vi "Magnet Test Communications.vi"(8 "error in (no error)":errorcluster, 11 "VISA resource name in":refnum<visa-resource-name>) -> (0 "error out":errorcluster, 3 "VISA resource name out":refnum<visa-resource-name>)   [LabVIEW 2016, in "Hall Effect Library.lvlib"]
uses:
  Hall Effect Library.lvlib
  Global Variables/Instruments.vi
  Magnet Test Communications (Manual).vi
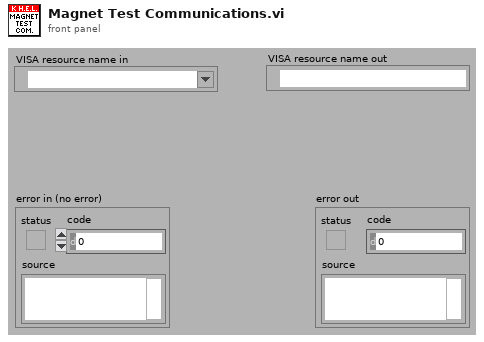
[diagram p1: front panel]
types:
  T1 = typedef "Hall Effect Library.lvlib/Magnets.ctl" = enum16{"Manual"}
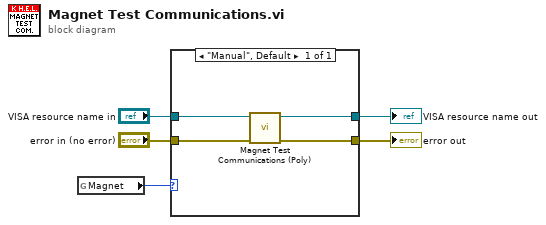
[diagram p0: block diagram]
diagram:
  n1 = global read "Instruments.vi" "Magnet"() -> (w5:T1)
  n2 = case shown="\"Manual\", Default" w5 {
    tunnel: "error in (no error)" -> [w9]
    tunnel: [w8] -> w2
    tunnel: [w7] -> w1
    tunnel: "VISA resource name in" -> [w6]
    frame "Manual", Default {
      n3 = call-poly "Magnet Test Communications (Poly).vi"("error in (no error)"=w9, "VISA resource name in"=w6) -> ("error out"=w8:errorcluster, "VISA resource name out"=w7:refnum<visa-resource-name>)  [unwired: 8 out]
    }
  }
  "error out" <- w2
  "VISA resource name out" <- w1
